vi "Autotest_Instr.vi"(8 "error in (no error)":errorcluster caption="entrée d'erreur (pas d'erreur)", 11 "Class Instrument Multimeter en entrée":refnum<class "Class Instrument Schielding_Box.lvclass">) -> (0 "error out":errorcluster caption="sortie d'erreur", 3 "Class Instrument Multimeter en sortie":refnum<class "Class Instrument Schielding_Box.lvclass">)   [LabVIEW 2020, in "Library Instrument & Equipement.lvlib" / "Library Instruments.lvlib" / "Class Instrument Schielding_Box.lvclass"]
uses:
  Class Instrument Schielding_Box.lvclass
  C:/Users/ngarcin/OneDrive - Altyor/Standard TB/Class/Instrument/Instrument (Default)/Class Instrument (Default).lvclass
  Class Instrument Schielding_Box.lvclass/Class Instrument Schielding_Box.ctl
  Instrument (Default)/Class Instrument (Default).lvclass
  Shielding box/Class Shielding box (Default)/Class Shielding_ Box (Default).lvclass
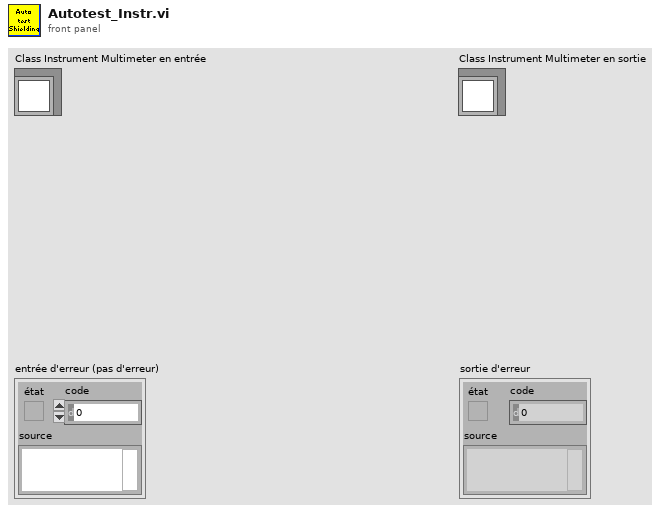
[diagram p1: front panel]
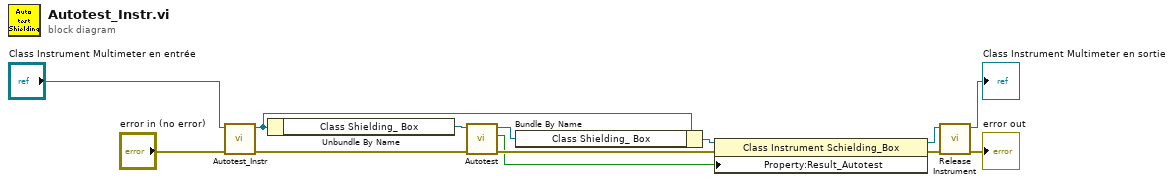
[diagram p0: block diagram]
diagram:
  n1 = call-parent "Autotest_Instr.vi"("error in (no error)"="error in (no error)", "Class Instrument (Default) en entrée"="Class Instrument Multimeter en entrée") -> ("error out"=w5:errorcluster, "Class Instrument (Default) en sortie"=w11:refnum<class "Class Instrument Schielding_Box.lvclass">)  [unwired: 8 in]
  n2 = Unbundle By Name(w11) -> ("Class Shielding_ Box"=w4:refnum<class "Class Shielding_ Box (Default).lvclass">)
  n3 = call-dynamic "Autotest.vi"("error in (no error)"=w5, "Class Shielding_ Box (Default) en entrée"=w4) -> ("error out"=w2:errorcluster, "Autotest Ok"=w1:bool, "Class Shielding_ Box (Default) en sortie"=w3:refnum<class "Class Shielding_ Box (Default).lvclass">)  [unwired: 7 in]
  n4 = Bundle By Name(cluster=w11, "Class Shielding_ Box"=w3) -> (w10:refnum<class "Class Instrument Schielding_Box.lvclass">)
  n5 = property class="Class Instrument Schielding_Box"(reference=w10, error in=w2, "Property:Result_Autotest"=w1) -> (reference out=w7:refnum<class "Class Instrument Schielding_Box.lvclass">, error out=w9:errorcluster)
  n6 = call-dynamic "Release Instrument.vi"("error in (no error)"=w9, "Class Instrument (Default) en entrée"=w7) -> ("error out"=→"error out":errorcluster, "Class Instrument (Default) en sortie"=→"Class Instrument Multimeter en sortie":refnum<class "Class Instrument Schielding_Box.lvclass">)  [unwired: 8 in]
